vi "Get Category.vi"(8 "error in (no error)":errorcluster, 11 "TEC editor node in":refnum<class "TEC editor node.lvclass">) -> (0 "error out":errorcluster, 2 "Category":string, 3 "TEC editor node out":refnum<class "TEC editor node.lvclass">)   [LabVIEW 2013, in "TEC editor node.lvclass"]
uses:
  TEC editor node.lvclass
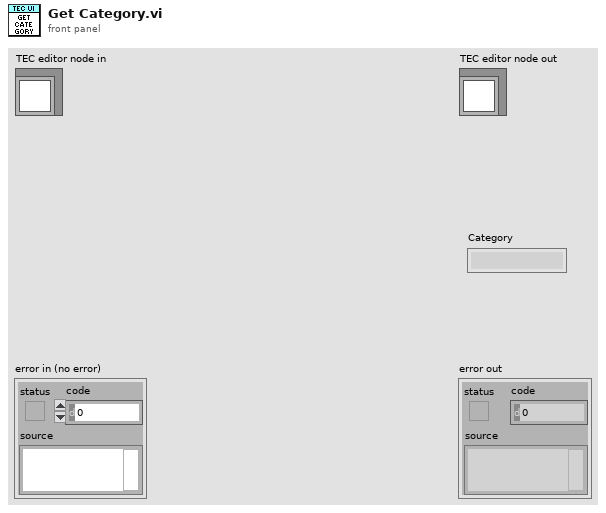
[diagram p1: front panel]
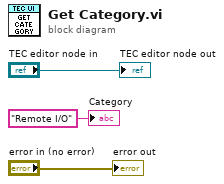
[diagram p0: block diagram]
diagram:
  "error out" <- "error in (no error)"
  "TEC editor node out" <- "TEC editor node in"
  "Category" <- "Remote I/O" ("Category")
